vi "Secure Client Connection.vi"(0 "TCP connection":refnum<k5>, 2 "certificate":u8[](array[numeric]), 4 "server hostname":string, 5 "error in":errorcluster, 8 "Secure the Connection (T)":bool=TRUE, 9 "load OS trusted CAs?":bool, 10 "timeout (25000 ms)":i32=25000, 11 "server certificate validation":enum32{"Any Trusted CA", "None"}(ring)) -> (14 "TCP connection out":refnum<k5>, 18 "server certificate chain":cluster{"certificate":u8[]}[](array[cluster]), 19 "error out":errorcluster)   [LabVIEW 2021, in "LV WebSockets.lvlib"]
doc: "Configures and negotiates a TLS client connection"
uses:
  LV WebSockets.lvlib
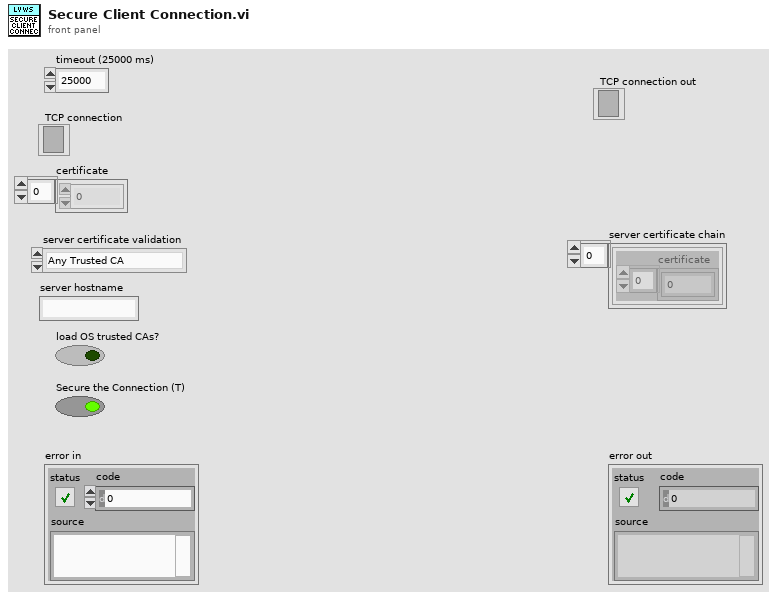
[diagram p1: front panel]
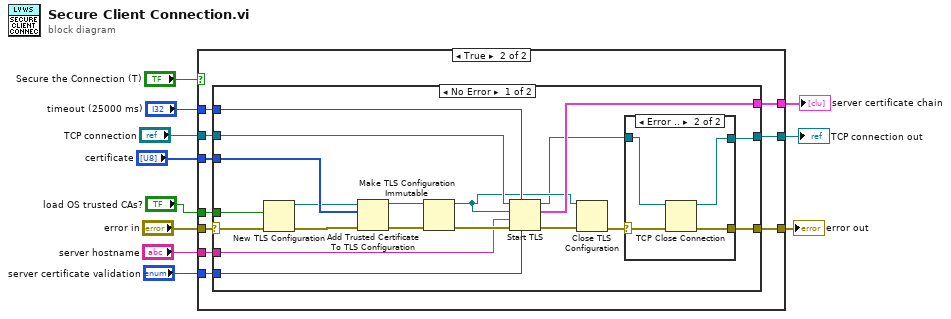
[diagram p0: block diagram]
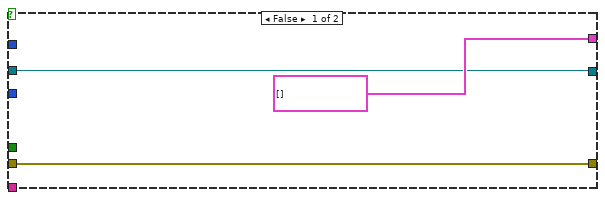
[diagram p2: hidden frame]
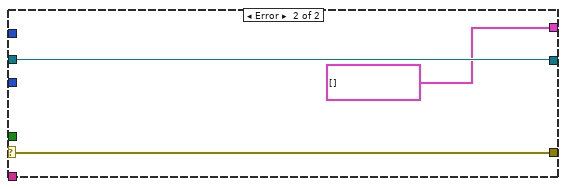
[diagram p4: hidden frame]
diagram:
  n1 = case shown="True" "Secure the Connection (T)" {
    tunnel: "certificate" -> [_ w24]
    tunnel: "timeout (25000 ms)" -> [_ w23]
    tunnel: "server certificate validation" -> [_ w22]
    tunnel: "server hostname" -> [_ w21]
    tunnel: "TCP connection" -> [w12 w20]
    tunnel: [cluster{"certificate":u8[]}[] [] ("server certificate chain") w19] -> w6
    tunnel: "error in" -> [w14 w18]
    tunnel: "load OS trusted CAs?" -> [_ w17]
    tunnel: [w14 w16] -> w3
    tunnel: [w12 w15] -> w2
    frame False {
    }
    frame True {
      n2 = case shown="No Error" w18 {
        selector: w18 -> [w34 w52]
        tunnel: w24 -> [w41 _]
        tunnel: w23 -> [w40 _]
        tunnel: w22 -> [w39 _]
        tunnel: w21 -> [w37 _]
        tunnel: w20 -> [w36 w51]
        tunnel: [w35 cluster{"certificate":u8[]}[] [] ("server certificate chain")] -> w19
        tunnel: w17 -> [w31 _]
        tunnel: [w26 w52] -> w16
        tunnel: [w25 w51] -> w15
        frame No Error {
          n3 = New TLS Configuration(8:w34, 10:w31) -> (0:w33:errorcluster, 3:w32:refnum<k36>)
          n4 = Add Trusted Certificate To TLS Configuration(8:w33, 10:w41, 11:w32) -> (0:w42:errorcluster, 3:w43:refnum<k36>)
          n5 = Make TLS Configuration Immutable(8:w42, 11:w43) -> (0:w38:errorcluster, 3:w29:refnum<k36>)
          n6 = Start TLS(6:w39, 7:w40, 8:w38, 9:w37, 10:w29, 11:w36) -> (0:w30:errorcluster, 2:w35:cluster{"certificate":u8[]}[], 3:w27:refnum<k5>)
          n7 = Close TLS Configuration(8:w30, 11:w29) -> (0:w28:errorcluster)
          n8 = case shown="Error .." w28 {
            selector: w28 -> [w45 w49]
            tunnel: w27 -> [w44 w47]
            tunnel: [w45 w48] -> w26
            tunnel: [w44 w46] -> w25
            frame No Error {
            }
            frame Error {
              n9 = TCP Close Connection(connection ID=w47, error in (no error)=w49) -> (connection ID out=w46:refnum<k5>, error out=w48:errorcluster)  [unwired: 1 in]
            }
          }
        }
        frame Error {
        }
      }
    }
  }
  "server certificate chain" <- w6
  "error out" <- w3
  "TCP connection out" <- w2
